vi "Close Multipart Upload Reference.vi"(8 "error in (no error)":errorcluster, 11 "Multipart Upload RefNum in":T1) -> (0 "error out":errorcluster)   [LabVIEW 2015, in "LV Interface for Amazon S3.lvlib"]
doc: "This operation <B>closes the Multipart Upload Refnum</B>, so LabVIEW is able <B>to free up the resources allocated</B> during the upload process."
uses:
  LV Interface for Amazon S3.lvlib
  Typedefs/AMZ_S3_Multipart Upload RefNum.ctl
  Typedefs/AMZ_S3_Multipart Upload RefNum Enum.ctl
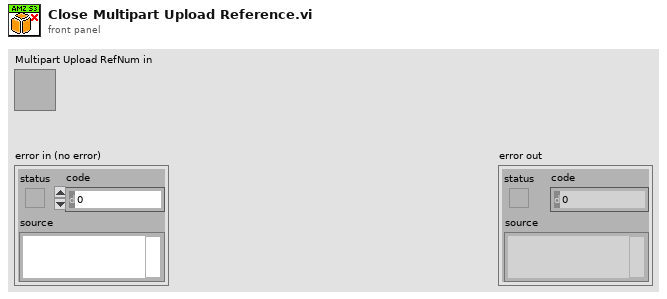
[diagram p1: front panel]
types:
  T1 = typedef "LV Interface for Amazon S3.lvlib/AMZ_S3_Multipart Upload RefNum.ctl" = refnum<k1>
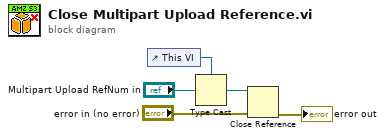
[diagram p0: block diagram]
diagram:
  n1 = control-ref of="This VI"() -> (w4:refnum<vi>)
  n2 = Type Cast(type=w4, x="Multipart Upload RefNum in") -> (*(type *) &x=w3:refnum<vi>)
  n3 = Close Reference(reference=w3, error in (no error)="error in (no error)") -> (error out=→"error out":errorcluster)
